vi "Robot.vi"() -> ()   [LabVIEW 2016]
uses:
  <vilib>/NXT/Subs/LVHSConnector.ctl
  <vilib>/NXT/LegoClasses/BrickReference/BrickReference.lvclass
  <vilib>/NXT/Block Support/NXT_InputPort.ctl
  <vilib>/NXT/Block Support/NXT_OutputPort.ctl
  <vilib>/NXT/Subs/ColorSensorColors.ctl
panel:
  out "Mode":dbl
  in  "Color \nSensor Port":T1=2 items=["Port 1", "Port 2", "Port 3", "Port 4"]
  in  "Enable State change":bool=TRUE
  in  "Motors 2":T2=7 items=["Port A", "Port B", "Port C", "Port D"]
  in  "Motors":T2=7 items=["Port A", "Port B", "Port C", "Port D"]
  in  "Kp":i32=1
  in  "Motor speed":i32=60
  in  "Gyro Port":T1 items=["Port 1", "Port 2", "Port 3", "Port 4"]
  in  "Distance to street":dbl
  in  "Sensor - Right":T1=3 items=["Port 1", "Port 2", "Port 3", "Port 4"]
  in  "Sensor - Left":T1=3 items=["Port 1", "Port 2", "Port 3", "Port 4"]
  in  "Colors and Directions":enum16{"Zero", "Right", "Front", "Left"}[](array[ring])=[enum."Zero", enum."Zero", enum."Zero", enum."Zero", enum."Zero", enum."Zero"]
  in  "Correct":bool
  in  "CS":T3(ring)
  out "NXT/EV3 2":T4
  in  "NXT/EV3":T4
  # "Blue"
  # "Green"
  # "Red"
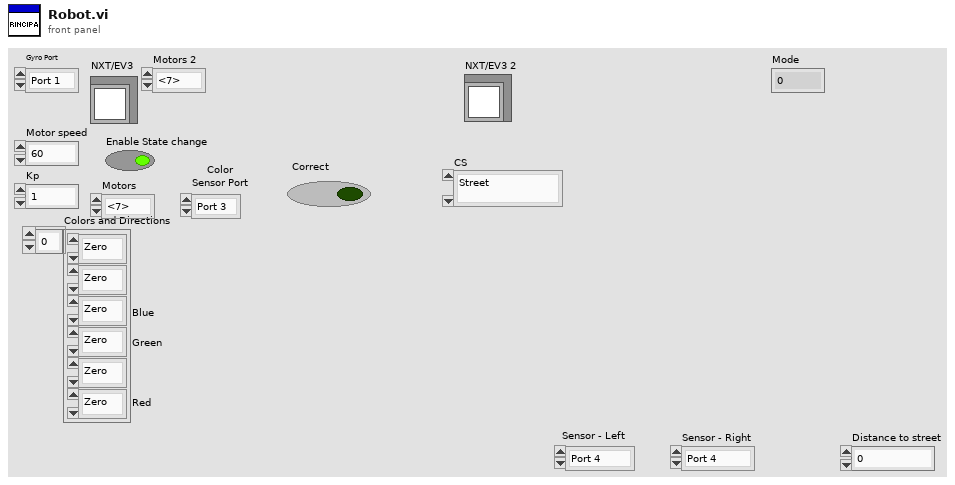
[diagram p1: front panel]
types:
  T1 = typedef "NXT_InputPort.ctl" = u32
  T2 = typedef "NXT_OutputPort.ctl" = u8
  T3 = enum16{"Street", "Intersection", "End", "Stop", "Square", "Delivery"}
  T4 = typedef "LVHSConnector.ctl" = refnum<class "BrickReference.lvclass">
  T5 = typedef "ColorSensorColors.ctl" = enum16{"No Color", "Black", "Blue", "Green", "Yellow", "Red", "White", "Brown"}
  T6 = enum16{"Street", "Intersection", "End", "Stop", "Square"}
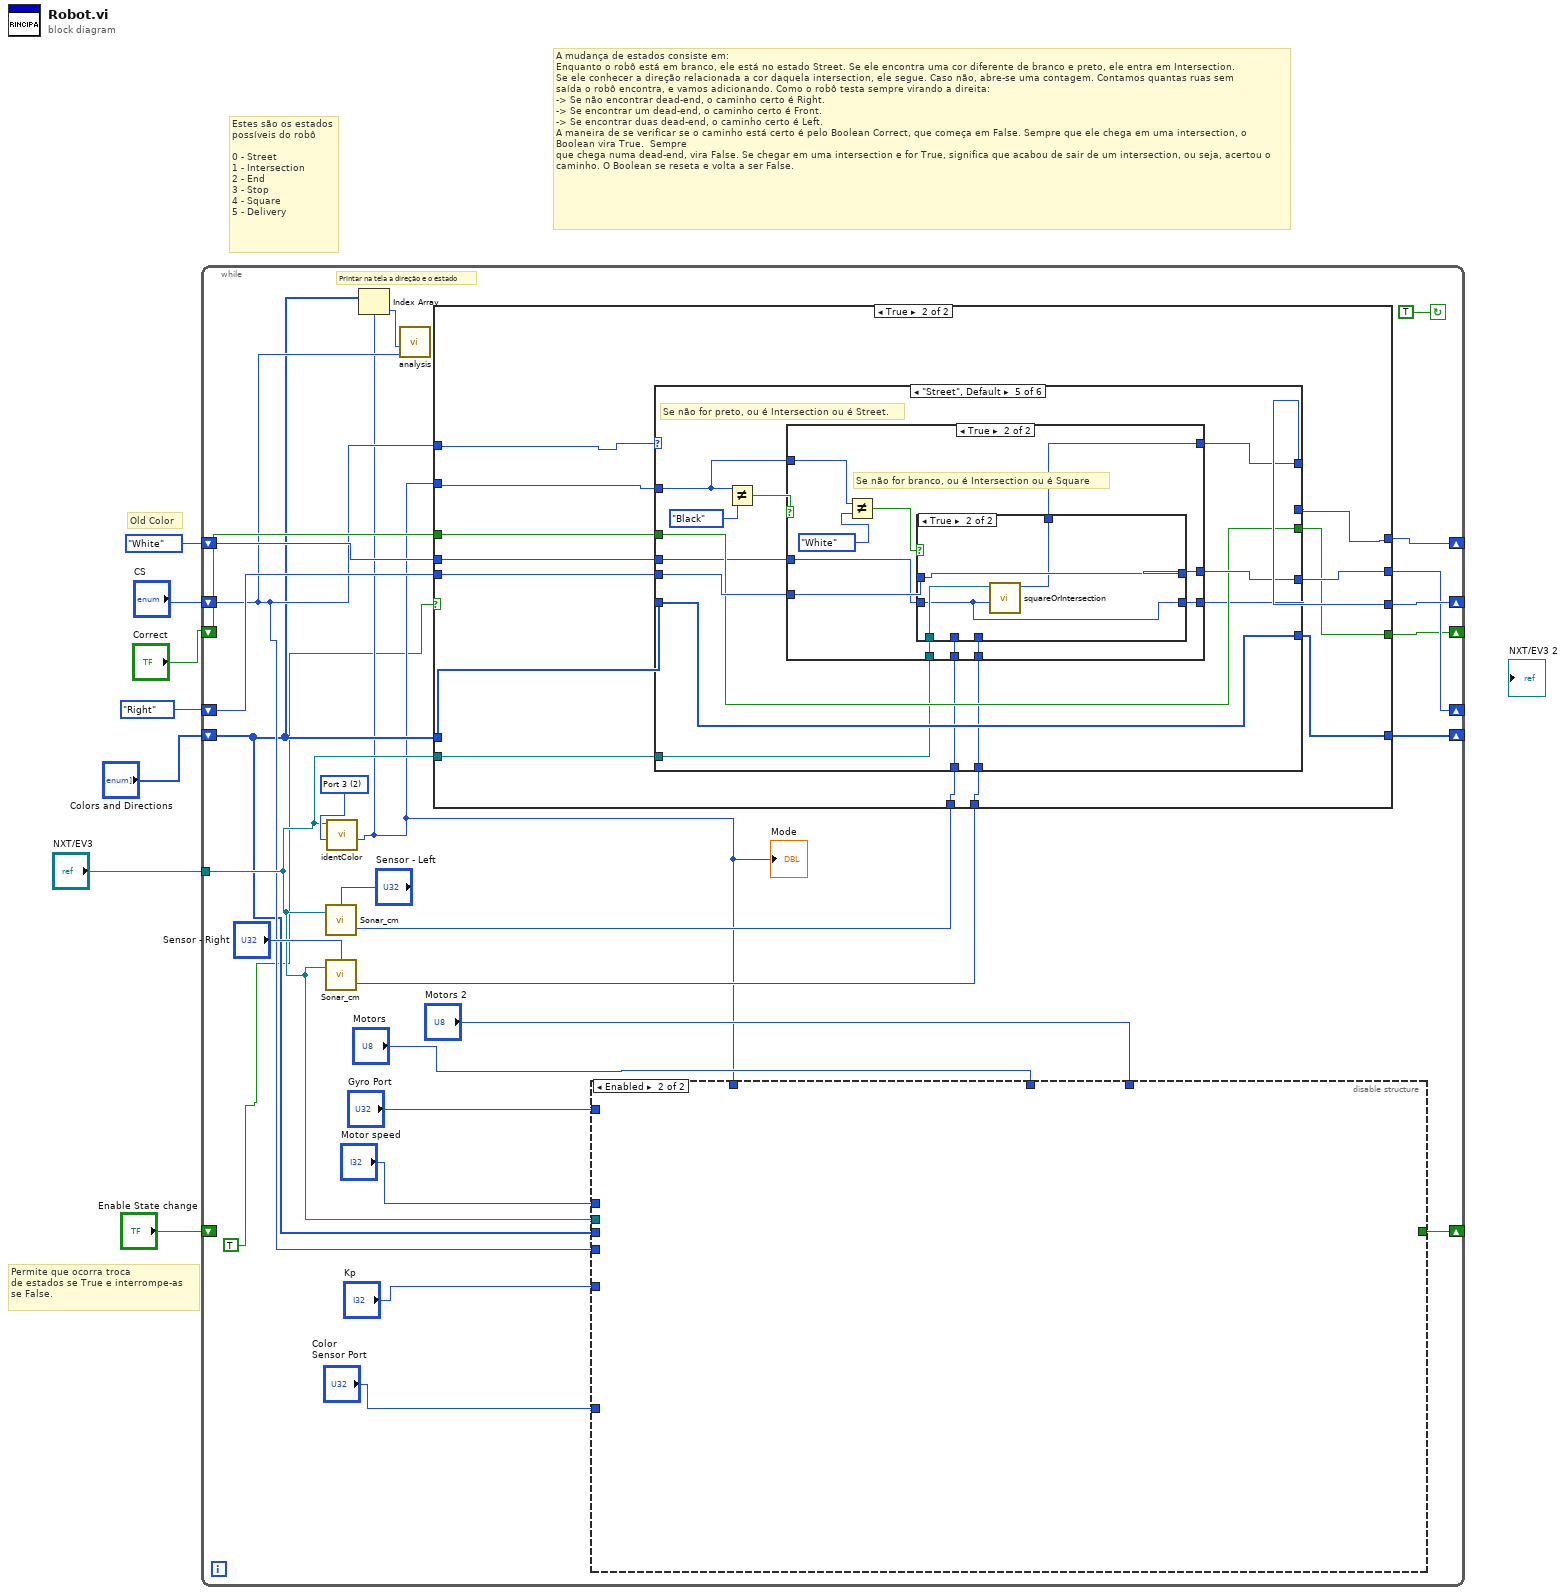
[diagram p0: block diagram]
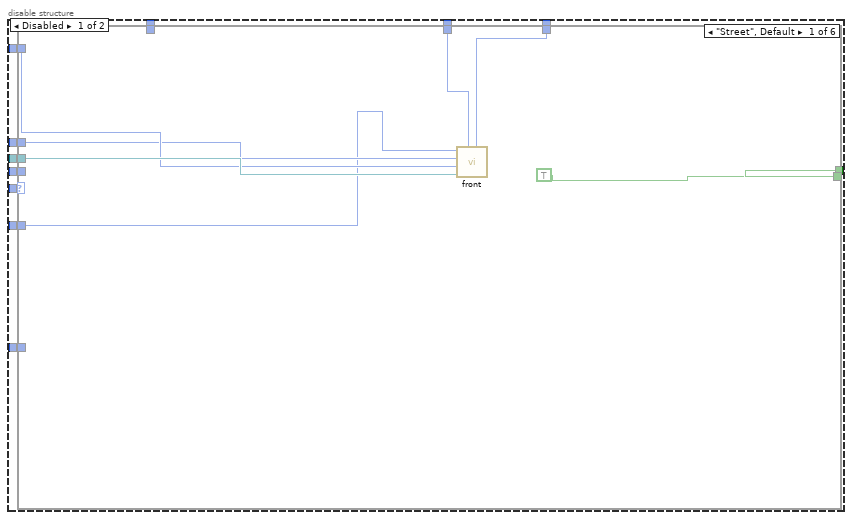
[diagram p2: hidden frame]
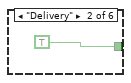
[diagram p3: hidden frame]
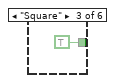
[diagram p4: hidden frame]
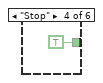
[diagram p5: hidden frame]
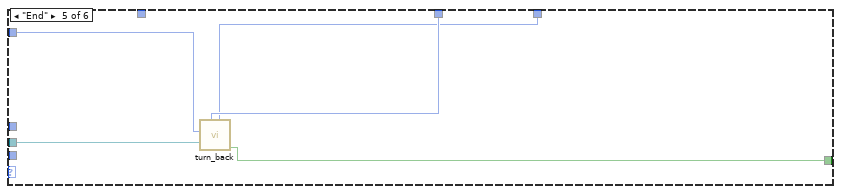
[diagram p6: hidden frame]
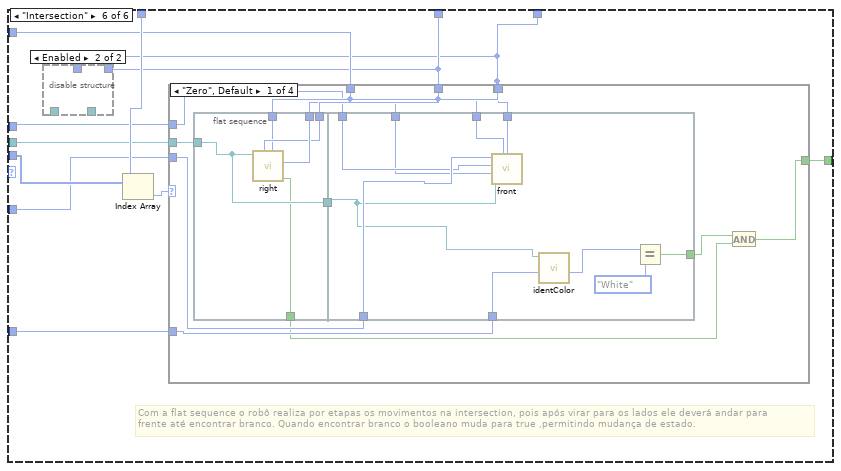
[diagram p7: hidden frame]
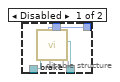
[diagram p8: hidden frame]
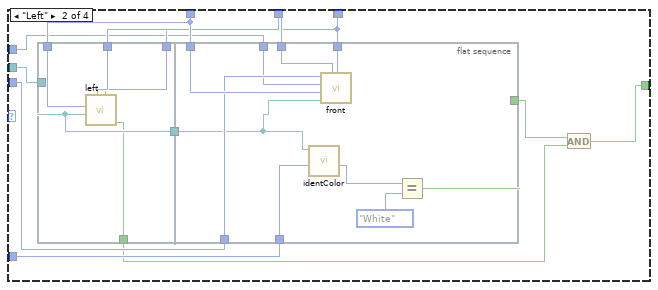
[diagram p9: hidden frame]
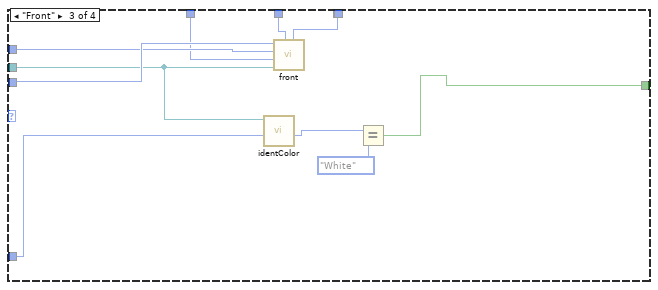
[diagram p10: hidden frame]
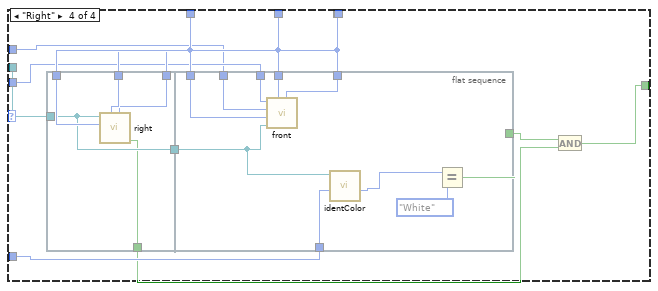
[diagram p11: hidden frame]
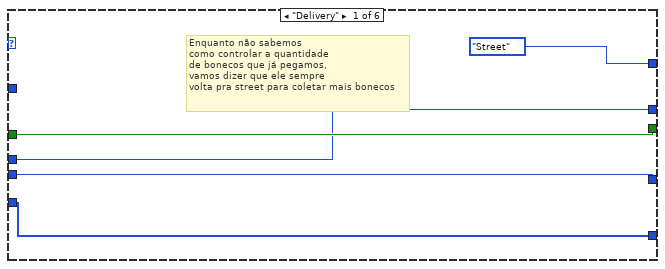
[diagram p13: hidden frame]
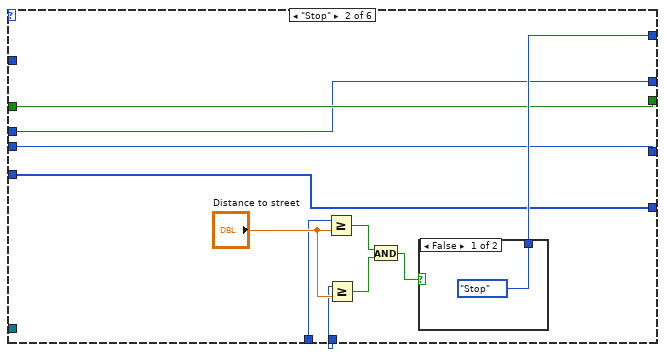
[diagram p14: hidden frame]
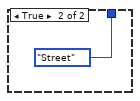
[diagram p15: hidden frame]
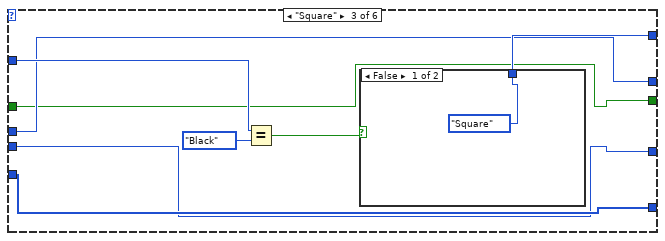
[diagram p16: hidden frame]
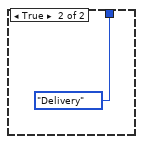
[diagram p17: hidden frame]
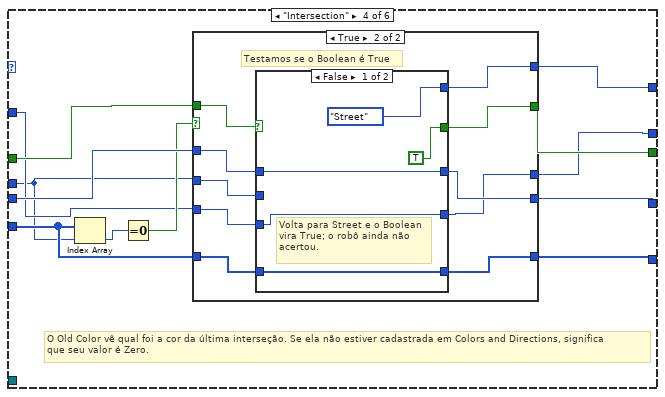
[diagram p18: hidden frame]
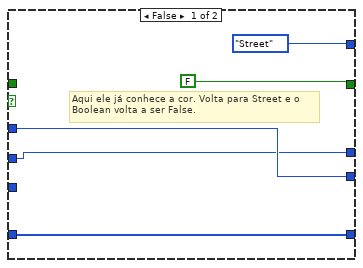
[diagram p19: hidden frame]
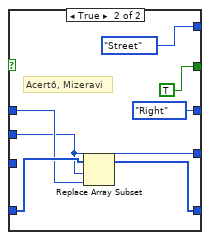
[diagram p20: hidden frame]
diagram:
  # "Permite que ocorra troca \nde estados se True e interrompe-as \nse False."
  # "A mudança de estados consiste em:\nEnquanto o robô está em branco, ele está no estado Street. Se ele encontra uma cor diferente de branco e preto, ele entra em Intersection.\nSe ele conhecer a direção relacionada a cor daquela intersection, ele segue. Caso não, abre-se uma contagem. Contamos quantas ruas sem \nsaída o robô encontra, e vamos adicionando. Como o robô testa sempre virando a direita:\n-> Se não encontrar dead-end, o caminho certo é Right.\n-> Se encontrar um dead-end, o caminho certo é Front.\n-> Se encontrar duas dead-end, o caminho certo é Left.\nA maneira de se verificar se o caminho está certo é pelo Boolean Correct, que começa em False. Sempre que ele chega em uma intersection, o Boolean vira True.  Sempre\nque chega numa dead-end, vira False. Se chegar em uma intersection e for True, significa que acabou de sair de um intersection, ou seja, acertou o\ncaminho. O Boolean se reseta e volta a ser False."
  # "Estes são os estados\npossíveis do robô\n\n0 - Street\n1 - Intersection\n2 - End\n3 - Stop\n4 - Square\n5 - Delivery"
  # "Old Color"
  n1 = while {
    tunnel: "NXT/EV3" -> [w14]
    shift-right: [w33] -> _
    shift-left: "CS" -> [w13]
    shift-right: [w31] -> _
    shift-left: enum16{"Zero", "Right", "Front", "Left"}."Right" ("Direction") -> [w32]
    shift-right: [w29] -> _
    shift-left: "Correct" -> [w30]
    shift-right: [w9] -> _
    shift-left: "Colors and Directions" -> [w12]
    shift-right: [w28] -> _
    shift-left: ColorSensorColors."White" ("Detected Color") -> [w27]
    shift-right: [w17] -> _
    shift-left: "Enable State change" -> [_]
    stop <- TRUE continue-if-true
    w15 = T1 2 items=["Port 1", "Port 2", "Port 3", "Port 4"] ("Port (Port 3)")
    # "Printar na tela a direção e o estado"
    n2 = call <vilib>:"Sonar_cm.vi"("NXT/EV3"=w14, "Port (Port 4)"="Sensor - Left") -> ("Distance (cm)"=w24:i16)  [unwired: 1 in, 1 out]
    n3 = call <vilib>:"Sonar_cm.vi"("NXT/EV3"=w14, "Port (Port 4)"="Sensor - Right") -> ("Distance (cm)"=w23:i16)  [unwired: 1 in, 1 out]
    n4 = call "identColor.vi"("Port (Port 1)"=w15, "NXT/EV3"=w14) -> ("Collor"=w11:T5)  [unwired: 9 in]
    "Mode" <- w11
    n5 = Index Array(array=w12, index=w11) -> (element=w10:enum16{"Zero", "Right", "Front", "Left"})
    n6 = call "analysis.vi"("CS 2"=w13, "Direction"=w10) -> ()  [unwired: 10 in]
    n7 = case shown="True" TRUE {
      tunnel: [w168 w183] -> w33
      tunnel: w32 -> [w166 w182]
      tunnel: [w166 w181] -> w31
      tunnel: w30 -> [w167 w180]
      tunnel: [w167 w179] -> w29
      tunnel: [w169 w172] -> w28
      tunnel: w27 -> [w169 w171]
      tunnel: w24 -> [_ w178]
      tunnel: w23 -> [_ w177]
      tunnel: w13 -> [w168 w176]
      tunnel: w14 -> [_ w175]
      tunnel: w12 -> [w165 w174]
      tunnel: w11 -> [_ w170]
      tunnel: [w165 w173] -> w9
      frame False {
      }
      frame True {
        n8 = case shown="\"Street\", Default" w176 {
          tunnel: w170 -> [_ _ w208 w214 w260 _]
          tunnel: [enum16{"Street", "Intersection", "End", "Stop"}."Street" ("CS") w193 w206 w221 w263 enum16{"Street", "Intersection", "End"}."Street" ("CS")] -> w183
          tunnel: w182 -> [w185 w189 w204 w219 w259 w289]
          tunnel: [w185 w189 w204 w220 w258 w289] -> w181
          tunnel: w180 -> [w187 w192 w202 w223 w256 _]
          tunnel: [w187 w192 w202 w222 w256 FALSE] -> w179
          tunnel: w174 -> [w184 w191 w205 w215 w257 w291]
          tunnel: [w184 w191 w205 w216 w257 w291] -> w173
          tunnel: [w186 w190 w203 w212 w251 w290] -> w172
          tunnel: w171 -> [w186 w190 w203 w213 w252 w290]
          tunnel: w178 -> [_ w198 _ _ w255 _]
          tunnel: w177 -> [_ w197 _ _ w254 _]
          tunnel: w175 -> [_ _ _ _ w253 _]
          frame "Delivery" {
            # "Enquanto não sabemos\ncomo controlar a quantidade\nde bonecos que já pegamos,\nvamos dizer que ele sempre\nvolta pra street para coletar mais bonecos"
          }
          frame "Stop" {
            n9 = Greater Or Equal?(x=w198, y="Distance to street") -> (x >= y?=w195:bool)
            n10 = Greater Or Equal?(x=w197, y="Distance to street") -> (x >= y?=w196:bool)
            n11 = And(x=w195, y=w196) -> (x .and. y?=w194:bool)
            n12 = case shown="False" w194 {
              tunnel: [enum16{"Street", "Intersection", "End", "Stop"}."Stop" ("CS") enum16{"Street", "Intersection", "End", "Stop"}."Street" ("CS")] -> w193
              frame False {
              }
              frame True {
              }
            }
          }
          frame "Square" {
            n13 = Equal?(x=w208, y=ColorSensorColors."Black") -> (x = y?=w207:bool)
            n14 = case shown="False" w207 {
              tunnel: [T3."Square" ("CS") T3."Delivery" ("CS")] -> w206
              frame False {
              }
              frame True {
              }
            }
          }
          frame "Intersection" {
            # "O Old Color vê qual foi a cor da última interseção. Se ela não estiver cadastrada em Colors and Directions, significa\nque seu valor é Zero."
            n15 = Index Array(array=w215, index=w213) -> (element=w218:enum16{"Zero", "Right", "Front", "Left"})
            n16 = Equal To 0?(x=w218) -> (x = 0?=w217:bool)
            n17 = case shown="True" w217 {
              tunnel: w223 -> [_ w238]
              tunnel: [FALSE w237] -> w222
              tunnel: [enum16{"Street", "Intersection", "End"}."Street" ("CS") w236] -> w221
              tunnel: [w226 w235] -> w220
              tunnel: w219 -> [w226 w234]
              tunnel: [w227 w233] -> w216
              tunnel: w215 -> [w227 w232]
              tunnel: w214 -> [_ w231]
              tunnel: [w224 w229] -> w212
              tunnel: w213 -> [w224 w230]
              frame False {
                # "Aqui ele já conhece a cor. Volta para Street e o \nBoolean volta a ser False."
              }
              frame True {
                # "Testamos se o Boolean é True"
                n18 = case shown="False" w238 {
                  tunnel: [TRUE TRUE] -> w237
                  tunnel: [enum16{"Street", "Intersection", "End"}."Street" ("CS") enum16{"Street", "Intersection", "End"}."Street" ("CS")] -> w236
                  tunnel: [w241 enum16{"Zero", "Right", "Front", "Left"}."Right" ("Direction")] -> w235
                  tunnel: w234 -> [w241 w246]
                  tunnel: [w239 w245] -> w233
                  tunnel: w232 -> [w239 w247]
                  tunnel: w231 -> [w240 _]
                  tunnel: [w240 w244] -> w229
                  tunnel: w230 -> [_ w244]
                  frame False {
                    # "Volta para Street e o Boolean\nvira True; o robô ainda não\nacertou."
                  }
                  frame True {
                    # "Acertô, Mizeravi"
                    n19 = Replace Array Subset(array=w247, new element=w246, index=w244) -> (w245:enum16{"Zero", "Right", "Front", "Left"}[])
                  }
                }
              }
            }
          }
          frame "Street", Default {
            # "Se não for preto, ou é Intersection ou é Street."
            n20 = Not Equal?(x=w260, y=ColorSensorColors."Black" ("Detected Color")) -> (x != y?=w261:bool)
            n21 = case shown="True" w261 {
              tunnel: [enum16{"Street", "Intersection", "End"}."End" ("CS") w275] -> w263
              tunnel: w260 -> [_ w277]
              tunnel: w259 -> [w266 w274]
              tunnel: [w265 w273] -> w258
              tunnel: w255 -> [_ w272]
              tunnel: w254 -> [_ w271]
              tunnel: w253 -> [_ w270]
              tunnel: w252 -> [w264 w269]
              tunnel: [w264 w268] -> w251
              frame False {
                # "Nesse caso, ele chegou numa dead-end; vai para o estado End\ne adiciona um no contador."
                n22 = Increment(x=w266) -> (x+1=w265:enum16{"Zero", "Right", "Front", "Left"})
              }
              frame True {
                # "Se não for branco, ou é Intersection ou é Square"
                n23 = Not Equal?(x=w277, y=ColorSensorColors."White" ("Detected Color")) -> (x != y?=w276:bool)
                n24 = case shown="True" w276 {
                  tunnel: [w280 w285] -> w275
                  tunnel: w274 -> [w283 w287]
                  tunnel: [w283 w287] -> w273
                  tunnel: w272 -> [w282 _]
                  tunnel: w271 -> [w281 _]
                  tunnel: w270 -> [_ w286]
                  tunnel: w269 -> [w279 w284]
                  tunnel: [w279 w284] -> w268
                  frame False {
                    # "Ou ele vai para Stop ou continua em Street"
                    n25 = call "toStop.vi"("Left"=w282, "Right"=w281) -> ("Next State"=w280:enum16{"Street", "Intersection", "End", "Stop"})  [unwired: 13 in]
                  }
                  frame True {
                    n26 = call "squareOrIntersection.vi"("Old Color IN"=w284, "NXT/EV3"=w286) -> ("CS"=w285:T6)  [unwired: 9 in]
                  }
                }
              }
            }
          }
          frame "End" {
            # "Depois de um End, ele sempre volta para Street, e o Boolean vira False"
          }
        }
      }
    }
    n27 = disable-structure shown="Enabled" {
      disable-tunnel: "Gyro Port" -> [w45 _]
      disable-tunnel: "Motor speed" -> [w44 _]
      disable-tunnel: "Motors" -> [w43 _]
      disable-tunnel: "Motors 2" -> [w42 _]
      disable-tunnel: "Kp" -> [w41 _]
      disable-tunnel: [w40 _] -> w17
      disable-tunnel: "Color \nSensor Port" -> [w39 _]
      disable-tunnel: w14 -> [w38 _]
      disable-tunnel: w13 -> [w37 _]
      disable-tunnel: w12 -> [w36 _]
      disable-tunnel: w11 -> [w35 _]
      frame Disabled {
        n28 = case shown="\"Street\", Default" w37 {
          tunnel: w38 -> [w52 _ _ _ w60 w61]
          tunnel: w45 -> [w51 _ _ _ w57 w67]
          tunnel: w44 -> [w50 _ _ _ _ w68]
          tunnel: w43 -> [w49 _ _ _ w59 w66]
          tunnel: w42 -> [w48 _ _ _ w58 w64]
          tunnel: w36 -> [_ _ _ _ _ w71]
          tunnel: w35 -> [_ _ _ _ _ w70]
          tunnel: w41 -> [w47 _ _ _ _ w69]
          tunnel: [TRUE TRUE ("x = y?") TRUE ("x = y?") TRUE ("x = y?") w56 w65] -> w40
          tunnel: w39 -> [_ _ _ _ _ w63]
          frame "Street", Default {
            n29 = call "front.vi"("Motors 2"=w48, "Motors"=w49, "NXT/EV3"=w52, "Gyro Port"=w51, "Motor speed"=w50, "Kp"=w47) -> ()  [unwired: 6 in]
          }
          frame "Delivery" {
          }
          frame "Square" {
          }
          frame "Stop" {
          }
          frame "End" {
            n30 = call "turn_back.vi"("Motors 2"=w58, "Motors"=w59, "NXT/EV3"=w60, "Gyro Port"=w57) -> ("x = y?"=w56:bool)  [unwired: 7 in]
          }
          frame "Intersection" {
            # "Com a flat sequence o robô realiza por etapas os movimentos na intersection, pois após virar para os lados ele deverá andar para\nfrente até encontrar branco. Quando encontrar branco o booleano muda para true ,permitindo mudança de estado."
            n31 = disable-structure shown="Enabled" {
              disable-tunnel: _ -> [w75 _]
              disable-tunnel: [w74 _] -> _
              disable-tunnel: w66 -> [w73 _]
              disable-tunnel: w64 -> [w72 _]
              frame Disabled {
                n32 = call "brake.vi"("Motors 2"=w72, "Motors"=w73, "NXT/EV3"=w75) -> ("NXT/EV3 2"=w74:T4)  [unwired: 8 in]
              }
              frame Enabled {
              }
            }
            n33 = Index Array(array=w71, index=w70) -> (element=w62:enum16{"Zero", "Right", "Front", "Left"})
            n34 = case shown="\"Zero\", Default" w62 {
              tunnel: w61 -> [w87 w113 w130 w149]
              tunnel: w66 -> [w84 w110 w138 w146]
              tunnel: w64 -> [w86 w109 w137 w145]
              tunnel: w69 -> [w85 w108 w136 w144]
              tunnel: w68 -> [w82 w107 w135 w143]
              tunnel: w67 -> [w81 w111 w134 w147]
              tunnel: [w76 w103 w132 w139] -> w65
              tunnel: w64 -> [w83 _ _ _]
              tunnel: w63 -> [w79 w106 w131 w142]
              frame "Zero", Default {
                n35 = flat-sequence {
                  tunnel: w87 -> [w89]
                  tunnel: w81 -> [w92]
                  tunnel: w84 -> [w91]
                  tunnel: w86 -> [w90]
                  tunnel: [w89] -> w80
                  tunnel: [w88] -> w77
                  tunnel: w85 -> [w101]
                  tunnel: w84 -> [w100]
                  tunnel: w83 -> [w99]
                  tunnel: w82 -> [w98]
                  tunnel: w81 -> [w97]
                  tunnel: w80 -> [w94]
                  tunnel: [w96] -> w78
                  tunnel: w79 -> [w95]
                  frame #0 {
                    n36 = call "right.vi"("Motors 2"=w90, "Motors"=w91, "Gyro Port"=w92, "NXT/EV3"=w89) -> ("x = y?"=w88:bool)  [unwired: 7 in]
                  }
                  frame #1 {
                    n37 = call "front.vi"("Motors 2"=w99, "Motors"=w100, "NXT/EV3"=w94, "Gyro Port"=w97, "Motor speed"=w98, "Kp"=w101) -> ()  [unwired: 6 in]
                    n38 = call "identColor.vi"("Port (Port 1)"=w95, "NXT/EV3"=w94) -> ("Collor"=w93:T5)  [unwired: 9 in]
                    n39 = Equal?(x=w93, y=ColorSensorColors."White") -> (x = y?=w96:bool)
                  }
                }
                n40 = And(x=w78, y=w77) -> (x .and. y?=w76:bool)
              }
              frame "Left" {
                n41 = flat-sequence {
                  tunnel: w110 -> [w118]
                  tunnel: w109 -> [w117]
                  tunnel: w111 -> [w116]
                  tunnel: w113 -> [w115]
                  tunnel: [w115] -> w112
                  tunnel: [w114] -> w104
                  tunnel: [w122] -> w105
                  tunnel: w112 -> [w120]
                  tunnel: w111 -> [w128]
                  tunnel: w110 -> [w127]
                  tunnel: w109 -> [w126]
                  tunnel: w108 -> [w125]
                  tunnel: w107 -> [w124]
                  tunnel: w106 -> [w121]
                  frame #0 {
                    n42 = call "left.vi"("Motors 2"=w117, "Motors"=w118, "NXT/EV3"=w115, "Gyro Port"=w116) -> ("x = y?"=w114:bool)  [unwired: 7 in]
                  }
                  frame #1 {
                    n43 = call "identColor.vi"("Port (Port 1)"=w121, "NXT/EV3"=w120) -> ("Collor"=w119:T5)  [unwired: 9 in]
                    n44 = call "front.vi"("Motors 2"=w126, "Motors"=w127, "NXT/EV3"=w120, "Gyro Port"=w128, "Motor speed"=w124, "Kp"=w125) -> ()  [unwired: 6 in]
                    n45 = Equal?(x=w119, y=ColorSensorColors."White") -> (x = y?=w122:bool)
                  }
                }
                n46 = And(x=w105, y=w104) -> (x .and. y?=w103:bool)
              }
              frame "Front" {
                n47 = call "identColor.vi"("Port (Port 1)"=w131, "NXT/EV3"=w130) -> ("Collor"=w129:T5)  [unwired: 9 in]
                n48 = call "front.vi"("Motors 2"=w137, "Motors"=w138, "NXT/EV3"=w130, "Gyro Port"=w134, "Motor speed"=w135, "Kp"=w136) -> ()  [unwired: 6 in]
                n49 = Equal?(x=w129, y=ColorSensorColors."White") -> (x = y?=w132:bool)
              }
              frame "Right" {
                n50 = flat-sequence {
                  tunnel: w146 -> [w154]
                  tunnel: w145 -> [w153]
                  tunnel: w149 -> [w151]
                  tunnel: w147 -> [w152]
                  tunnel: [w151] -> w148
                  tunnel: [w150] -> w140
                  tunnel: [w158] -> w141
                  tunnel: w148 -> [w157]
                  tunnel: w147 -> [w164]
                  tunnel: w146 -> [w163]
                  tunnel: w145 -> [w162]
                  tunnel: w144 -> [w161]
                  tunnel: w143 -> [w160]
                  tunnel: w142 -> [w155]
                  frame #0 {
                    n51 = call "right.vi"("Motors 2"=w153, "Motors"=w154, "Gyro Port"=w152, "NXT/EV3"=w151) -> ("x = y?"=w150:bool)  [unwired: 7 in]
                  }
                  frame #1 {
                    n52 = call "front.vi"("Motors 2"=w162, "Motors"=w163, "NXT/EV3"=w157, "Gyro Port"=w164, "Motor speed"=w160, "Kp"=w161) -> ()  [unwired: 6 in]
                    n53 = call "identColor.vi"("Port (Port 1)"=w155, "NXT/EV3"=w157) -> ("Collor"=w156:T5)  [unwired: 9 in]
                    n54 = Equal?(x=w156, y=ColorSensorColors."White") -> (x = y?=w158:bool)
                  }
                }
                n55 = And(x=w141, y=w140) -> (x .and. y?=w139:bool)
              }
            }
          }
        }
      }
      frame Enabled {
      }
    }
  }
